vi "DSC Plotter.vi"() -> ()   [LabVIEW 2020]
uses:
  Time_Slot--Control.ctl
  <vilib>/lvdsc/historical/Read Traces (Numeric).vi
  <vilib>/lvdsc/NI_DSC.lvlib
  <vilib>/lvdsc/historical/Read Trace (Numeric).vi
  <userlib>/_OpenG.lib/array/array.llb/Index 1D Array Elements (String)__ogtk.vi
panel:
  in  "Tree":string[](tree)
  out "error out":errorcluster
  out "quality":i32[][](array[numeric])
  in  "options":T1={"interpolate data (F)"=TRUE, "extrapolate to now (F)"=FALSE, "remove data breaks (F)"=TRUE, "interpolation interval (1 s)"=1.0, "maintain trending info (T)"=FALSE} {"interpolation interval (1 s)" min=0.0 format="%0.2f"}
  out "empty?":bool
  out "Argument":string
  in  "Traces":T2(array[cluster])
  out "busy":bool
  out "Array 2":timestamp[](array[timestamp])
  out "Array":timestamp[](array[timestamp])
  out "time (s)":sgl
  out "Children Tags":string[](array[string])
  in  "Presets":u16(ring) items=["Select Preset", "Clear Chart", "Add New Preset"]
  in  "Tab Control":enum32{"Main", "Custom Time", "Settings"}(tab)
  in  "Time slots":T3=enum."8 Hours"
  in  "Seek Back Button":bool
  in  "Seek Forward Button":bool
  in  "Display Current":bool
  in  "time interval":T4 {"stop timestamp (now)" format="%<%X\n%x>T"; "start timestamp" format="%<%X\n%x>T"}
  in  "Display Chose Time Slot":bool
  in  "update rate(ms)":i32=10000
  in  "max points per trace (all)":i32=1000
  in  "OK":bool
  out "XY Graph":T5(graph)
  # "Time Window (drop down 1hr 1 day etc)\nchoose channel/s\npresets (inc time window and channels)\nExport to csv.\nLive mode return\nIf you select manual time interval shows that until live mode return button pressed\nwould be nice to have arrows to go back and forth in time."
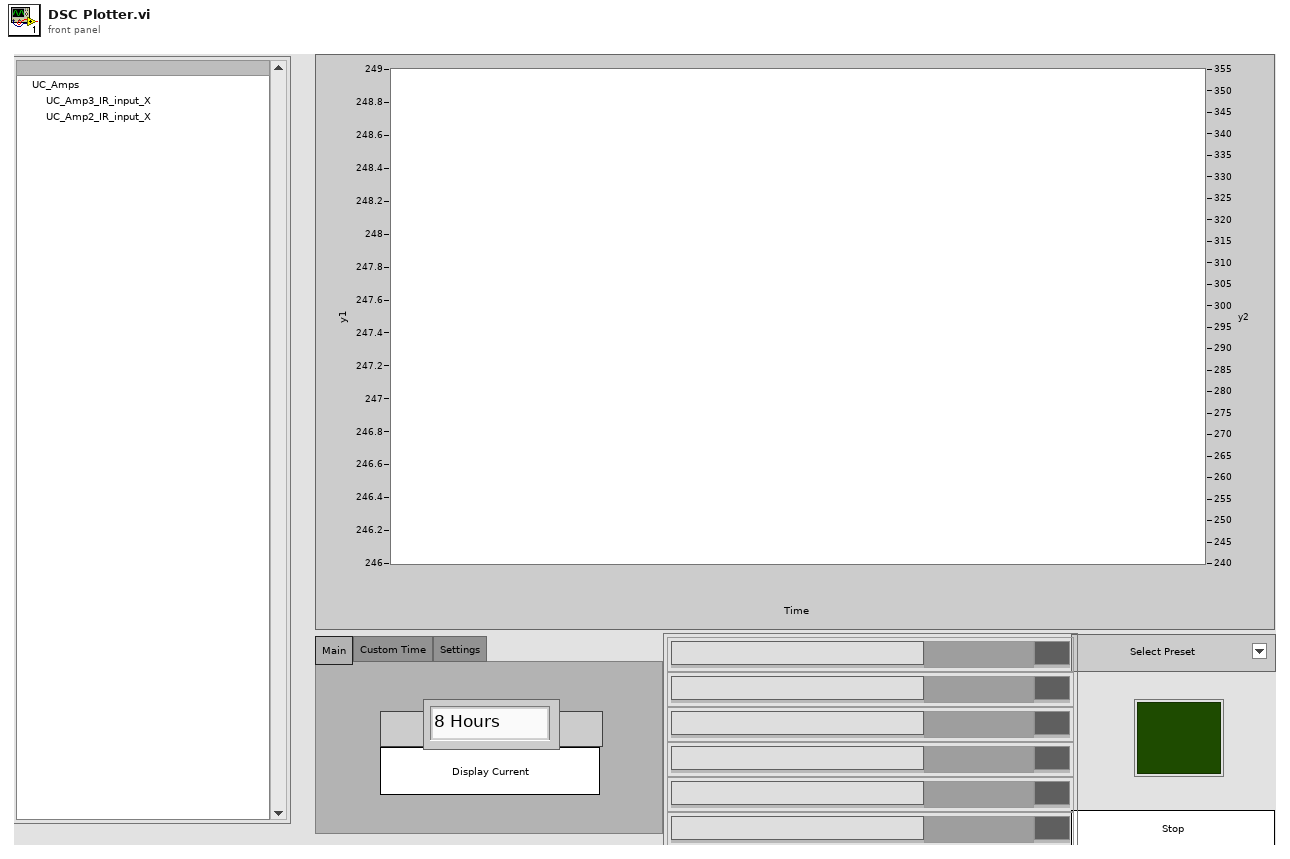
[diagram p1: front panel]
types:
  T1 = cluster{"interpolate data (F)":bool, "extrapolate to now (F)":bool, "remove data breaks (F)":bool, "interpolation interval (1 s)":dbl, "maintain trending info (T)":bool}
  T2 = cluster{"Name":string, "L/R scale":bool, "Color Box":u32}[]
  T3 = typedef "Time_Slot--Control.ctl" = enum16{"5 Mins", "15 Mins", "30 mins", "1 Hour", "8 Hours", "1 Day", "1 Week", "1 Month", "3 Months", "6 Months", "1 Year", "2 Years"}
  T4 = cluster{"start timestamp":timestamp, "stop timestamp (now)":timestamp}
  T5 = cluster{"timestamps":timestamp[], "data":dbl[]}[]
  T6 = cluster{"Name":string, "L/R scale":bool, "Color Box":u32}
  T7 = enum32{"invalid app kind", "Development System", "Run Time System", "Student Edition", "Embedded LabVIEW", "Evaluation", "Custom"}
  T8 = enum32{"Invalid", "Standard", "Closed", "Hidden", "Minimized", "Maximized"}
  T9 = cluster{"Core":cluster{"Current VI Reference":refnum<vi>, "Close Panel on Exit?":bool}, "options":cluster{"interpolate data (F)":bool, "extrapolate to now (F)":bool, "remove data breaks (F)":bool, "interpolation interval (1 s)":dbl, "maintain trending info (T)":bool}, "time interval":cluster{"start timestamp":timestamp, "stop timestamp (now)":timestamp}, "historical traces":cluster{"timestamps":timestamp[], "data":dbl[]}[], "Trace Names":string[], "max points per trace (all)":i32, "Time slots":T3, "Display Current Enable":bool, "update rate(ms)":i32, "All Traces from DB":string[], "Traces":cluster{"Name":string, "L/R scale":bool, "Color Box":u32}[]}
  T10 = typedef "mysql_authentication.ctl" = cluster{"User":string, "Password":string, "Database":string}
  T11 = cluster{"Port":u16, "IP Address":string, "Authentication":T10}
  T12 = cluster{"Current VI Reference":refnum<vi>, "Close Panel on Exit?":bool}
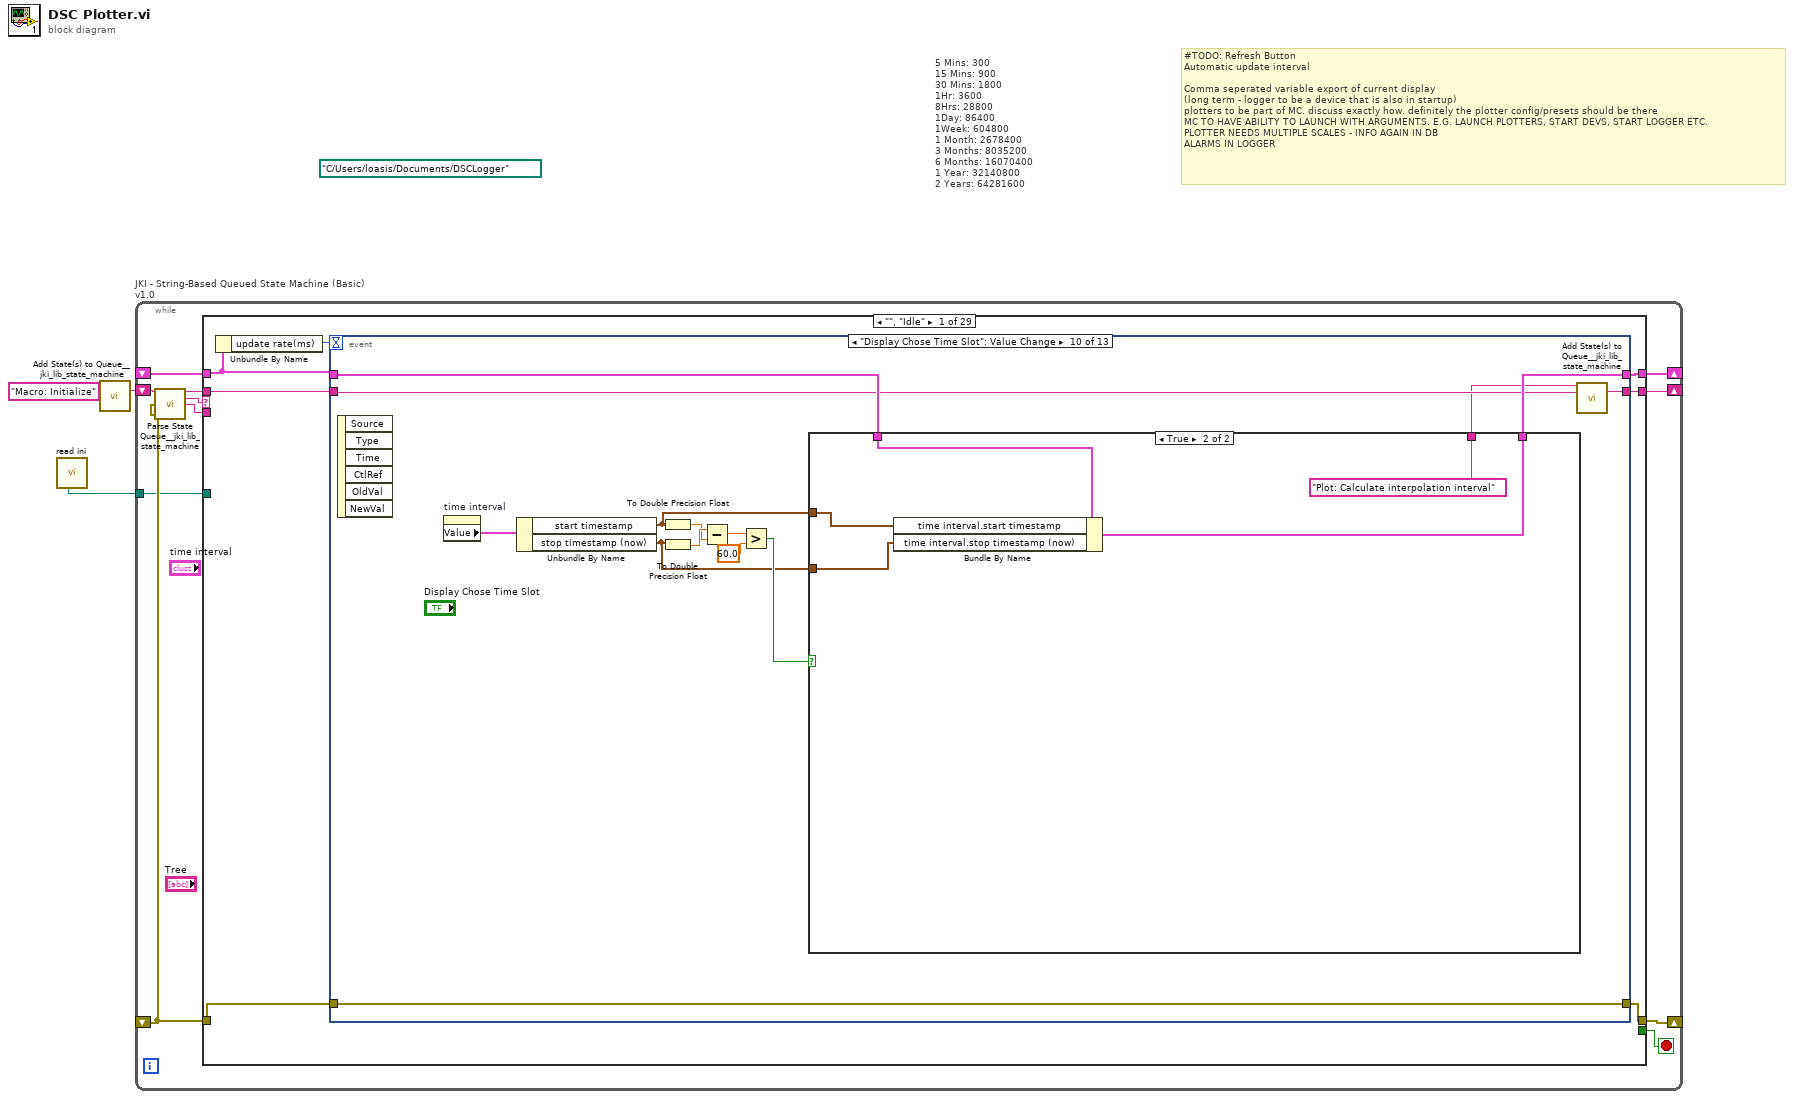
[diagram p0: block diagram]
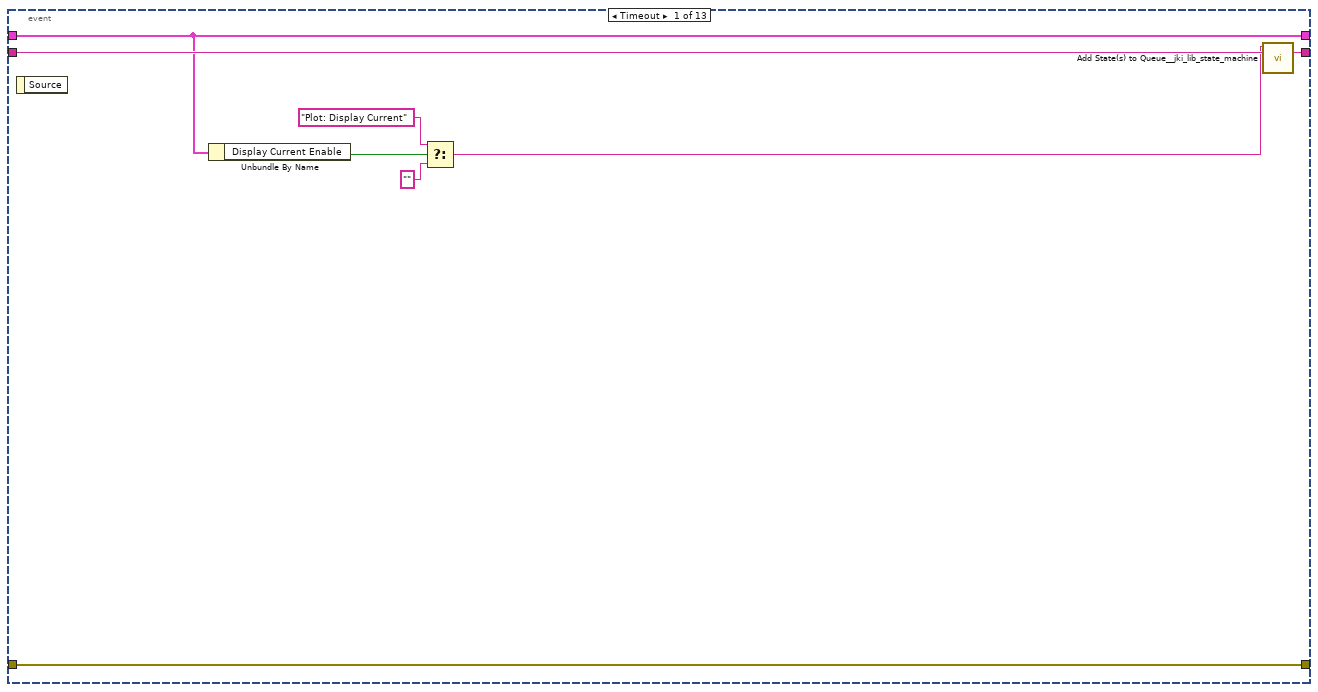
[diagram p2: hidden frame]
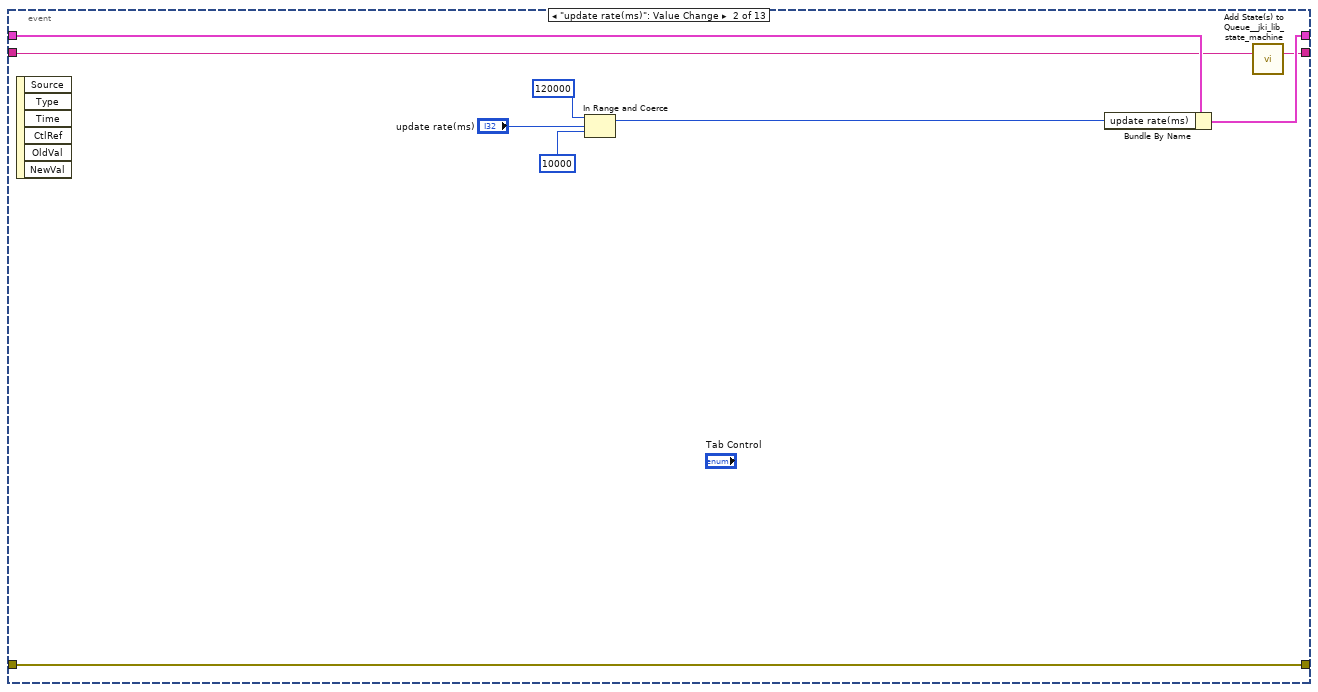
[diagram p3: hidden frame]
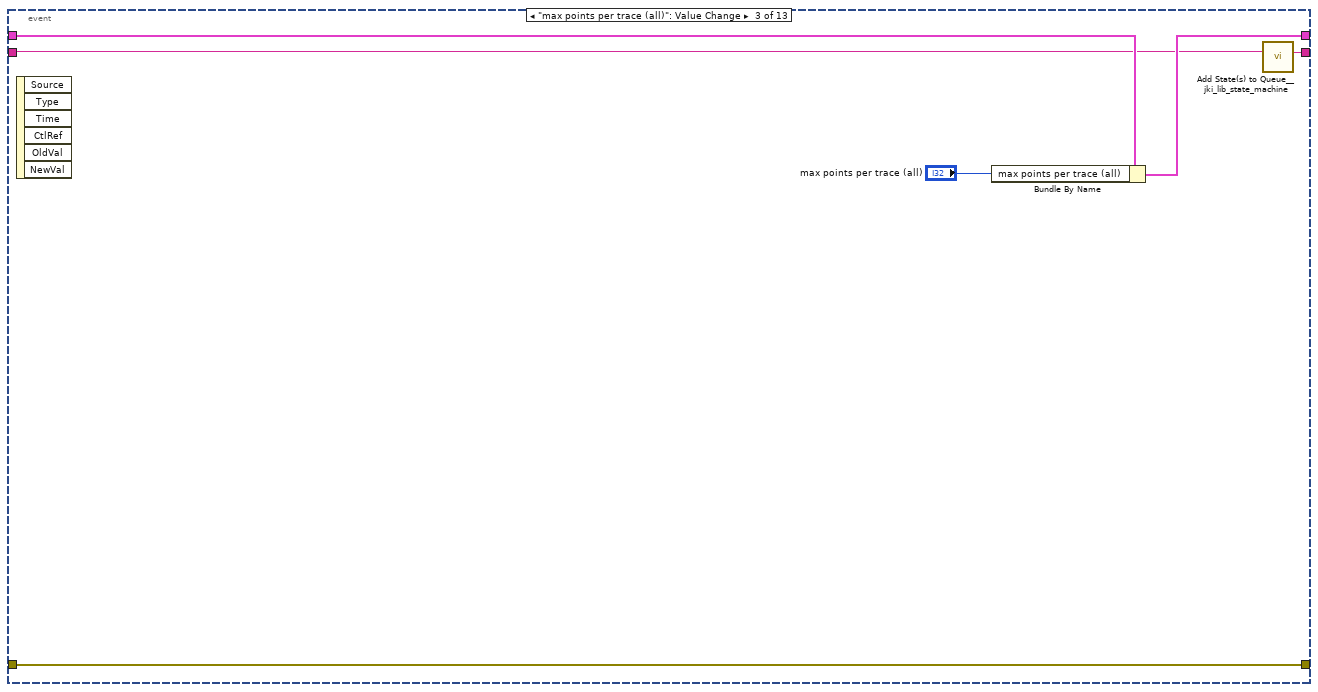
[diagram p4: hidden frame]
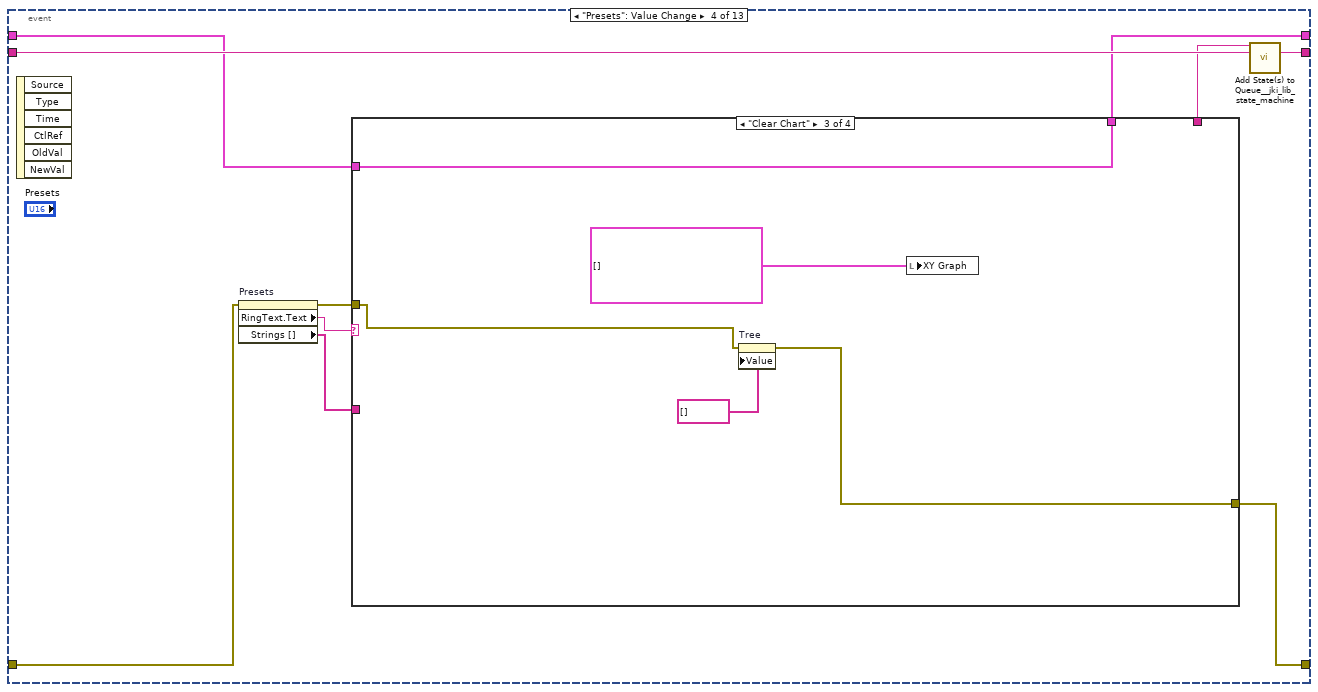
[diagram p5: hidden frame]
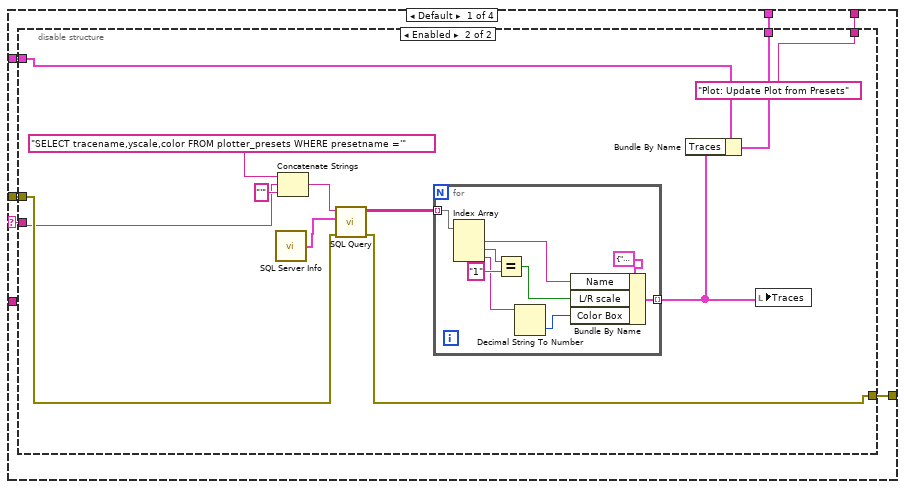
[diagram p6: hidden frame]
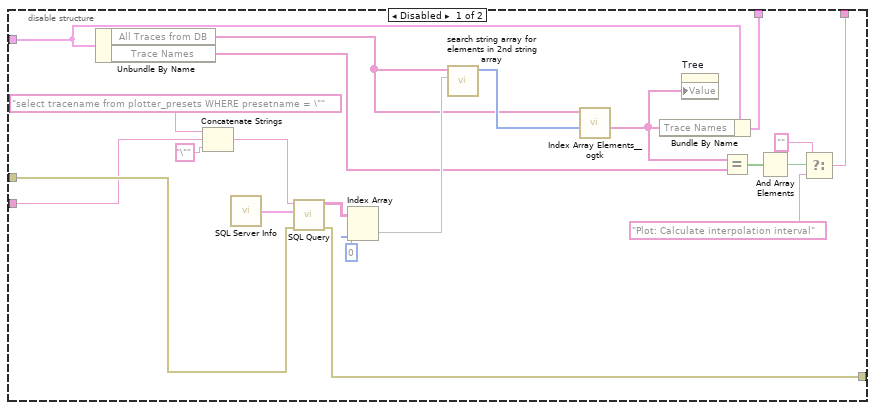
[diagram p7: hidden frame]
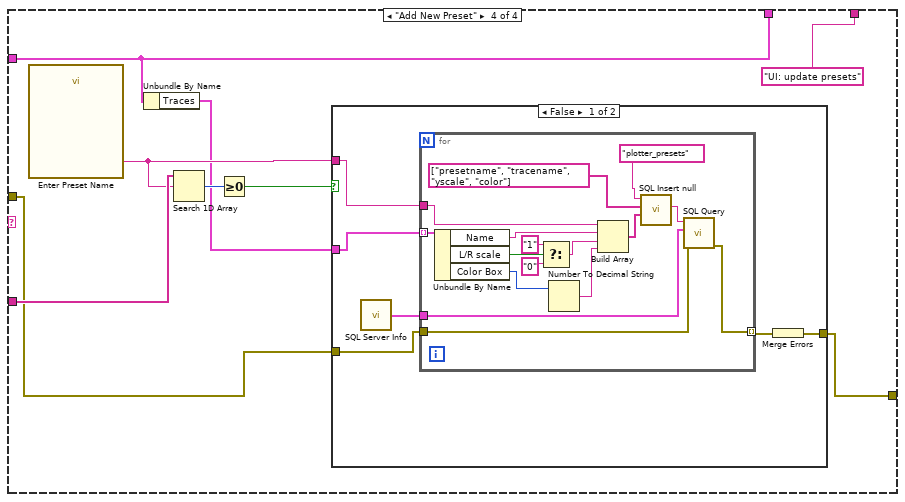
[diagram p9: hidden frame]
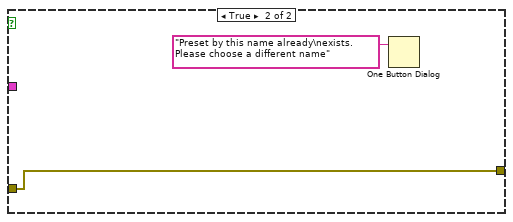
[diagram p10: hidden frame]
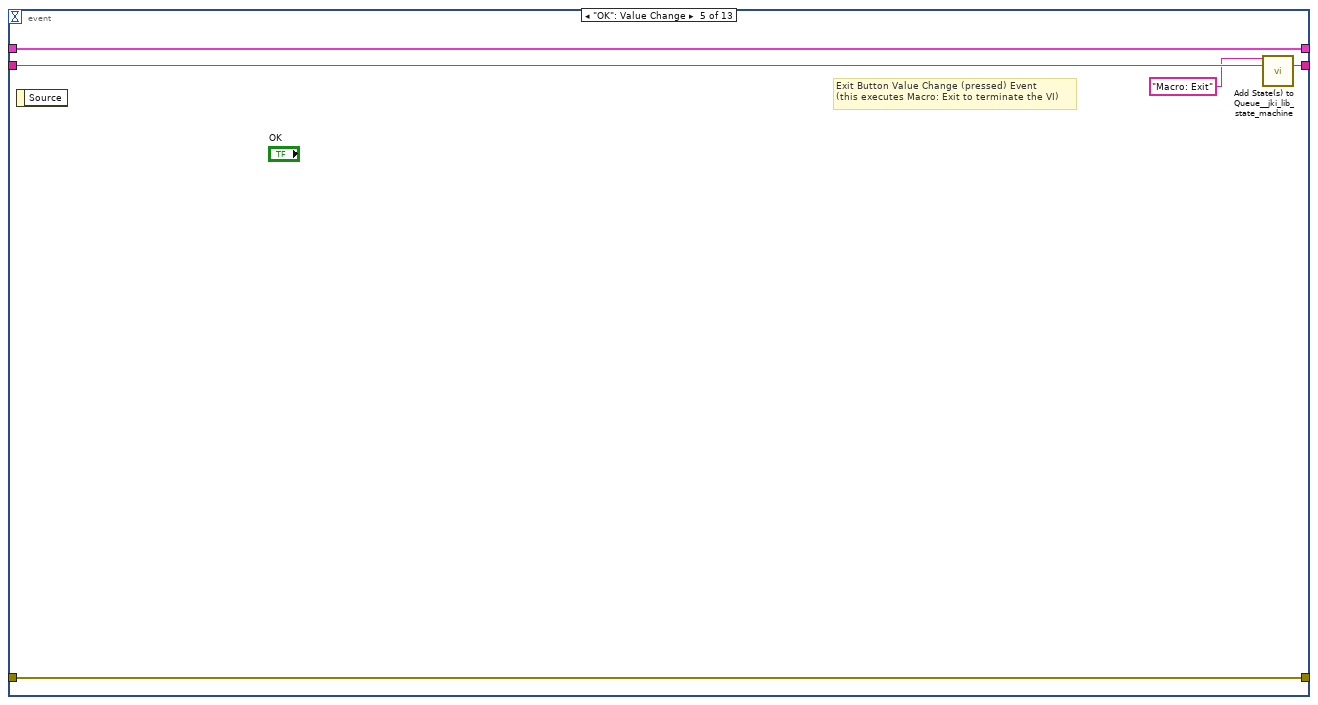
[diagram p11: hidden frame]
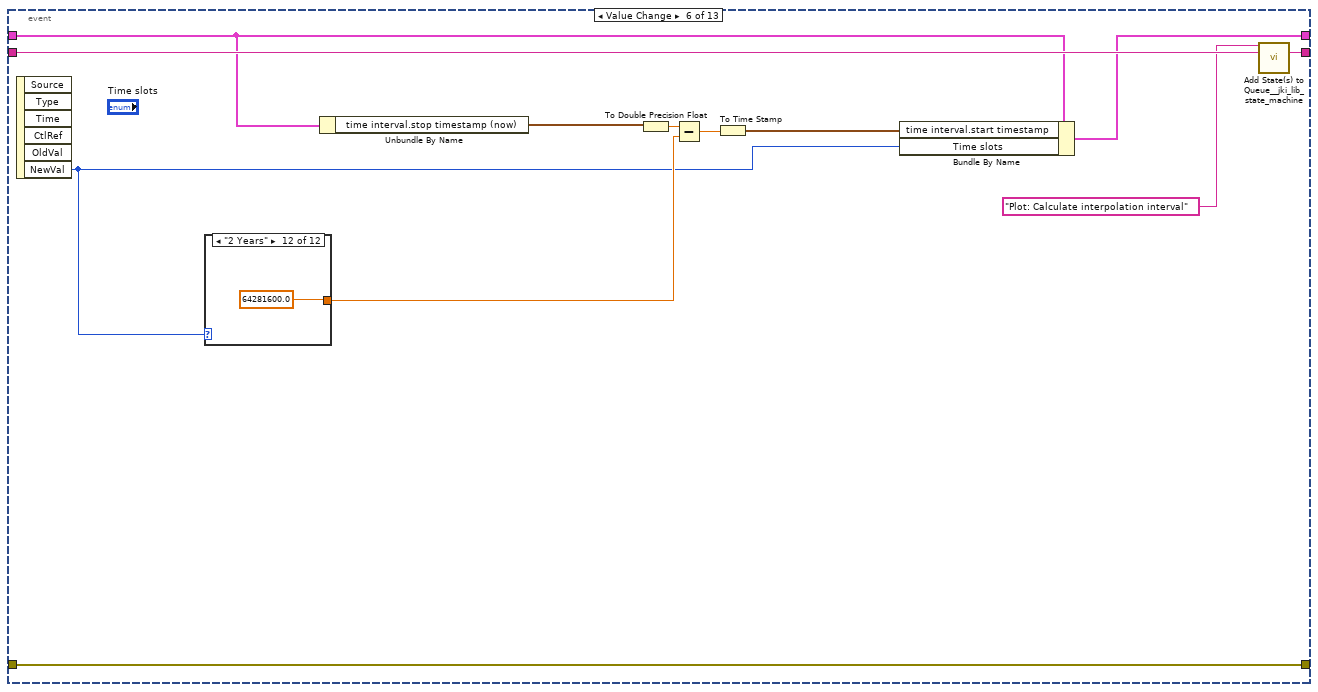
[diagram p12: hidden frame]
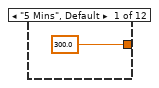
[diagram p13: hidden frame]
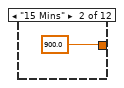
[diagram p14: hidden frame]
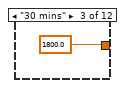
[diagram p15: hidden frame]
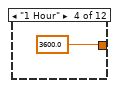
[diagram p16: hidden frame]
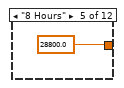
[diagram p17: hidden frame]
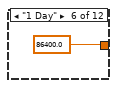
[diagram p18: hidden frame]
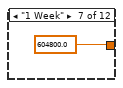
[diagram p19: hidden frame]
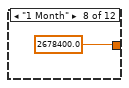
[diagram p20: hidden frame]
diagram:
  (unwired) path "C:/Users/loasis/Documents/DSCLogger" ("Application Directory")
  # "#TODO: Refresh Button\nAutomatic update interval\n\nComma seperated variable export of current display\n(long term - logger to be a device that is also in startup)\nplotters to be part of MC. discuss exactly how. definitely the plotter config/presets should be there\nMC TO HAVE ABILITY TO LAUNCH WITH ARGUMENTS. E.G. LAUNCH PLOTTERS, START DEVS, START LOGGER ETC.\nPLOTTER NEEDS MULTIPLE SCALES - INFO AGAIN IN DB\nALARMS IN LOGGER"
  # "5 Mins: 300\n15 Mins: 900\n30 Mins: 1800\n1Hr: 3600\n8Hrs: 28800\n1Day: 86400\n1Week: 604800\n1 Month: 2678400\n3 Months: 8035200\n6 Months: 16070400 \n1 Year: 32140800\n2 Years: 64281600"
  n1 = call "read ini.vi"() -> ("Database URL"=w1:path)  [unwired: 5 in, 6 out]
  n2 = call <vilib>:"Add State(s) to Queue__jki_lib_state_machine.vi"("State(s) in (\"\")"="Macro: Initialize") -> ("States Out"=w3:string)  [unwired: 14 in]
  n3 = while "JKI - String-Based Queued State Machine (Basic) v1.0" {
    shift-right: [w7] -> _
    shift-left: _ -> [w6]
    shift-right: [w10] -> _
    shift-left: _ -> [w5]
    shift-right: [w9] -> _
    shift-left: w3 -> [w11]
    tunnel: w1 -> [w4]
    stop <- w8 stop-if-true
    n4 = call <vilib>:"Parse State Queue__jki_lib_state_machine.vi"("State Queue"=w11, "Error In (no error)"=w5) -> ("Remaining States"=w13:string, "Current State"=w14:string, "Arguments"=w12:string)  [unwired: 11 in]
    n5 = case shown="\"\", \"Idle\"" w14 {
      selector: w14 -> [_ _ w348 _ _ _ _ _ _ _ _ _ _ _ _ _ _ _ _ _ _ _ _ _ _ _ _ _ _]
      tunnel: w13 -> [w21 w347 w352 w370 w376 w381 w385 w406 w412 w416 w431 w444 w472 w488 w499 w525 w530 w540 w544 w548 w553 w570 w579 w602 w623 w732 w749 w760 w770]
      tunnel: w12 -> [_ _ _ _ _ _ _ _ _ _ _ _ _ w483 w493 _ _ _ _ _ _ _ _ w589 w604 w726 _ _ _]
      tunnel: w6 -> [w16 w344 w350 w361 w373 w379 w382 _ w407 w413 w429 w442 w474 w486 w495 w522 w527 w537 w541 w545 w550 w566 w575 w595 w619 w730 w747 w758 w765]
      tunnel: [w19 w345 w354 w367 errorcluster {"status"=FALSE, "code"=0, "source"=""} ("error out") w378 w383 w403 w408 w414 w417 w432 w467 w484 w496 w523 w528 w538 w542 w546 w551 w568 w577 w600 w609 w729 w746 w752 w766] -> w10
      tunnel: w5 -> [w18 w345 w353 w367 w372 w378 w383 w403 w409 w414 w418 w433 w468 w485 w497 w523 w528 w538 w542 w546 w551 w568 w577 w600 w613 w729 w746 w753 w762]
      tunnel: [w20 w346 w351 w369 w375 w380 w384 w405 w411 w415 w430 w443 w473 w487 w498 w524 w529 w539 w543 w547 w552 w569 w578 w601 w622 w731 w748 w759 w769] -> w9
      tunnel: [_ _ _ _ _ TRUE _ _ _ _ _ _ _ _ _ _ _ _ _ _ _ _ _ _ _ _ _ _ _] -> w8
      tunnel: [w17 w344 w350 w368 w373 w379 w382 w404 w407 w413 w429 w442 w474 w486 w495 w522 w527 w537 w541 w545 w550 w565 w574 w594 w618 w730 w747 w757 w764] -> w7
      tunnel: w4 -> [_ _ _ _ _ _ _ _ _ _ _ _ _ _ _ _ _ _ _ _ _ _ _ _ w603 _ _ _ _]
      frame "", "Idle" {
        n6 = Unbundle By Name(w16) -> ("update rate(ms)"=w15:i32)
        n7 = event shown="[9] \"Display Chose Time Slot\": Value Change" {
          selector: _ -> [_ _ _ _ _ _ _ _ _ _ _ _ _]
          dyn-events: _ -> [_ _ _ _ _ _ _ _ _ _ _ _ _]
          timeout: w15 -> [_ _ _ _ _ _ _ _ _ _ _ _ _]
          tunnel: w21 -> [w29 w30 w39 w49 w147 w157 w174 w190 w209 w252 w285 w314 w343]
          tunnel: [w28 w31 w40 w50 w146 w158 w175 w191 w210 w253 w286 w315 w342] -> w20
          tunnel: w16 -> [w26 w37 w44 w48 w144 w153 w172 w183 w208 w257 w277 w306 w340]
          tunnel: [w27 w32 w41 w51 w145 w159 w176 w192 w211 w250 w287 w316 w341] -> w19
          tunnel: w18 -> [w27 w32 w41 w54 w145 w159 w176 w192 w211 w250 w287 w316 w341]
          tunnel: [w26 w38 w43 w47 w144 w152 w172 w189 w208 w254 w276 w305 w340] -> w17
          event Timeout {
            n8 = event-data() -> ()  [unwired: 1 in, 1 out]
            n9 = Unbundle By Name(w26) -> ("Display Current Enable"=w25:bool)
            n10 = Select(t="Plot: Display Current" ("State(s) in Front (\"\")"), s=w25, f="" ("State(s) in Front (\"\")")) -> (s? t:f=w23:string)
            n11 = call <vilib>:"Add State(s) to Queue__jki_lib_state_machine.vi"("State(s) in Front (\"\")"=w23, "State(s) in (\"\")"=w29) -> ("States Out"=w28:string)  [unwired: 13 in]
          }
          event "update rate(ms)": Value Change {
            n12 = event-data() -> ()  [unwired: 1 in, 6 out]
            n13 = In Range and Coerce(upper limit=120000, x="update rate(ms)", lower limit=10000) -> (coerced(x)=w33:i32)  [unwired: 1 out]
            n14 = Bundle By Name(cluster=w37, "update rate(ms)"=w33) -> (w38:T9)
            n15 = call <vilib>:"Add State(s) to Queue__jki_lib_state_machine.vi"("State(s) in (\"\")"=w30) -> ("States Out"=w31:string)  [unwired: 14 in]
          }
          event "max points per trace (all)": Value Change {
            n16 = event-data() -> ()  [unwired: 1 in, 6 out]
            n17 = Bundle By Name(cluster=w44, "max points per trace (all)"="max points per trace (all)") -> (w43:T9)
            n18 = call <vilib>:"Add State(s) to Queue__jki_lib_state_machine.vi"("State(s) in (\"\")"=w39) -> ("States Out"=w40:string)  [unwired: 14 in]
          }
          event "Presets": Value Change {
            n19 = event-data() -> ()  [unwired: 1 in, 6 out]
            n20 = property on="Presets" class="Ring (strict)"(error in=w54) -> (error out=w52:errorcluster, "RingText.Text"=w53:string, "Strings []"=w45:string[])  [unwired: 1 in, 1 out]
            n21 = case shown="\"Clear Chart\"" w53 {
              selector: w53 -> [w58 _ _ _]
              tunnel: w52 -> [w60 w103 w105 w114]
              tunnel: [w59 w103 w106 w113] -> w51
              tunnel: w48 -> [w57 w104 w109 w112]
              tunnel: [w56 w104 w109 w112] -> w47
              tunnel: [w55 _ _ "UI: update presets" ("t")] -> w46
              tunnel: w45 -> [_ _ _ w118]
              frame Default {
                n22 = disable-structure shown="Enabled" {
                  disable-tunnel: w60 -> [w80 w88]
                  disable-tunnel: [w79 w87] -> w59
                  disable-tunnel: w58 -> [w78 w86]
                  disable-tunnel: w57 -> [w69 w84]
                  disable-tunnel: [w68 w85] -> w56
                  disable-tunnel: [w62 "Plot: Update Plot from Presets" ("t")] -> w55
                  frame Disabled {
                    n23 = Unbundle By Name(w69) -> ("All Traces from DB"=w70:string[], "Trace Names"=w67:string[])
                    n24 = Concatenate Strings("select tracename from plotter_presets WHERE presetname = \"", w78, "\"" ("string")) -> (w76:string)
                    n25 = call "SQL Server Info.vi"() -> ("SQL Server Info"=w81:T11)
                    n26 = call "SQL Query.vi"("error in (no error)"=w80, "SQL Server Info"=w81, "Query"=w76) -> ("error out"=w79:errorcluster, "data"=w74:string[][])  [unwired: 7 in]
                    n27 = Index Array(array=w74, index (col)=0 ("index (row)")) -> (element=w72:string[])  [unwired: 1 in]
                    n28 = call "search string array for elements in 2nd string array.vi"("search for"=w72, "search in"=w70) -> ("Indices of Elements"=w71:i32[])  [unwired: 9 in]
                    n29 = call-poly <userlib>:"Index Array Elements__ogtk.vi"("indices"=w71, "array"=w70) -> ("elements"=w61:string[])  [unwired: 9 in]
                    n30 = Bundle By Name(cluster=w69, "Trace Names"=w61) -> (w68:T9)
                    n31 = property on="Tree" class="Tree (strict)"("Value"=w61) -> ()  [unwired: 2 in, 2 out]
                    n32 = Equal?(x=w61, y=w67) -> (x = y?=w66:bool[])
                    n33 = And Array Elements(Boolean array=w66) -> (logical AND=w65:bool)
                    n34 = Select(t="", s=w65, f="Plot: Calculate interpolation interval") -> (s? t:f=w62:string)
                  }
                  frame Enabled {
                    n35 = call "SQL Server Info.vi"() -> ("SQL Server Info"=w91:T11)
                    n36 = Concatenate Strings("SELECT tracename,yscale,color FROM plotter_presets WHERE presetname ='" ("Query"), w86, "'" ("string")) -> (w93:string)
                    n37 = call "SQL Query.vi"("error in (no error)"=w88, "SQL Server Info"=w91, "Query"=w93) -> ("error out"=w87:errorcluster, "data"=w89:string[][])  [unwired: 7 in]
                    n38 = for {
                      tunnel: w89 -> [w101] mode=indexing
                      tunnel: [w94] -> w83 mode=indexing
                      n39 = Index Array(array=w101) -> (element #1=w100:string, element #2=w99:string, element #3=w95:string)  [unwired: 3 in]
                      n40 = Equal?(x=w99, y="1") -> (x = y?=w97:bool)
                      n41 = Decimal String To Number(string=w95) -> (number=w96:i32)  [unwired: 2 in, 1 out]
                      n42 = Bundle By Name(cluster=T6 {"Name"="", "L/R scale"=FALSE, "Color Box"=0} ("Trace cluster"), "Name"=w100, "L/R scale"=w97, "Color Box"=w96) -> (w94:T6)
                    }
                    n43 = Bundle By Name(cluster=w84, "Traces"=w83) -> (w85:T9)
                    n44 = local write "Traces"(w83) -> ()
                  }
                }
              }
              frame "Select Preset" {
              }
              frame "Clear Chart" {
                n45 = property on="Tree" class="Tree (strict)"(error in=w105, "Value"=string[] [] ("Tree")) -> (error out=w106:errorcluster)  [unwired: 1 in, 1 out]
                n46 = local write "XY Graph"(T5 [] ("XY Graph")) -> ()
              }
              frame "Add New Preset" {
                n47 = call "Enter Preset Name"() -> ("Preset Name"=w115:string)  [unwired: 17 in, 2 out]
                n48 = Unbundle By Name(w112) -> ("Traces"=w111:T2)
                n49 = Search 1D Array(1D array=w118, element=w115) -> (index of element=w117:i32)  [unwired: 1 in]
                n50 = Greater Or Equal To 0?(x=w117) -> (x >= 0?=w116:bool)
                n51 = case shown="False" w116 {
                  tunnel: w111 -> [w123 _]
                  tunnel: w115 -> [w122 _]
                  tunnel: w114 -> [w121 w141]
                  tunnel: [w119 w141] -> w113
                  frame False {
                    n52 = call "SQL Server Info.vi"() -> ("SQL Server Info"=w124:T11)
                    n53 = for {
                      tunnel: w124 -> [w140]
                      tunnel: w123 -> [w132] mode=indexing
                      tunnel: w122 -> [w135]
                      tunnel: w121 -> [w134]
                      tunnel: [w133] -> w120 mode=indexing
                      n54 = Unbundle By Name(w132) -> ("Name"=w131:string, "L/R scale"=w130:bool, "Color Box"=w126:u32)
                      n55 = Select(t="1", s=w130, f="0") -> (s? t:f=w127:string)
                      n56 = Number To Decimal String(number=w126) -> (decimal integer string=w125:string)  [unwired: 1 in]
                      n57 = Build Array(w135, w131, w127, w125) -> (w136:string[])
                      n58 = call "SQL Insert null.vi"("Values"=w136, "Column Names"=string[] ["presetname", "tracename", "yscale", "color"], "Table"="plotter_presets") -> ("Query String"=w139:string)  [unwired: 8 in]
                      n59 = call "SQL Query.vi"("error in (no error)"=w134, "SQL Server Info"=w140, "Query"=w139) -> ("error out"=w133:errorcluster)  [unwired: 7 in, 1 out]
                    }
                    n60 = Merge Errors(w120) -> (w119:errorcluster)
                  }
                  frame True {
                    n61 = One Button Dialog(message="Preset by this name already\nexists. Please choose a different name") -> ()  [unwired: 1 in, 1 out]
                  }
                }
              }
            }
            n62 = call <vilib>:"Add State(s) to Queue__jki_lib_state_machine.vi"("State(s) in Front (\"\")"=w46, "State(s) in (\"\")"=w49) -> ("States Out"=w50:string)  [unwired: 13 in]
          }
          event "OK": Value Change {
            # "Exit Button Value Change (pressed) Event\n(this executes Macro: Exit to terminate the VI)"
            n63 = event-data() -> ()  [unwired: 1 in, 1 out]
            n64 = call <vilib>:"Add State(s) to Queue__jki_lib_state_machine.vi"("State(s) in Front (\"\")"="Macro: Exit", "State(s) in (\"\")"=w147) -> ("States Out"=w146:string)  [unwired: 13 in]
          }
          event Value Change {
            n65 = event-data() -> ("NewVal"=w148:T3)  [unwired: 1 in, 5 out]
            n66 = case shown="\"2 Years\"" w148 {
              tunnel: [300.0 ("y") 900.0 ("y") 1800.0 ("y") 3600.0 ("y") 28800.0 ("y") 86400.0 ("y") 604800.0 ("y") 2678400.0 ("y") 8035200.0 ("y") 16070400.0 ("y") 32140800.0 ("y") 64281600.0 ("y")] -> w154
              frame "5 Mins", Default {
              }
              frame "15 Mins" {
              }
              frame "30 mins" {
              }
              frame "1 Hour" {
              }
              frame "8 Hours" {
              }
              frame "1 Day" {
              }
              frame "1 Week" {
              }
              frame "1 Month" {
              }
              frame "3 Months" {
              }
              frame "6 Months" {
              }
              frame "1 Year" {
              }
              frame "2 Years" {
              }
            }
            n67 = Unbundle By Name(w153) -> ("time interval.stop timestamp (now)"=w155:timestamp)
            n68 = To Double Precision Float(number=w155) -> (double precision float=w156:dbl)
            n69 = Subtract(x=w156, y=w154) -> (x-y=w151:dbl)
            n70 = To Time Stamp(1:w151) -> (0:w150:timestamp)
            n71 = Bundle By Name(cluster=w153, "time interval.start timestamp"=w150, "Time slots"=w148) -> (w152:T9)
            n72 = call <vilib>:"Add State(s) to Queue__jki_lib_state_machine.vi"("State(s) in Front (\"\")"="Plot: Calculate interpolation interval" ("State(s) in Front (\"\")"), "State(s) in (\"\")"=w157) -> ("States Out"=w158:string)  [unwired: 13 in]
          }
          event "Display Current": Value Change {
            n73 = event-data() -> ()  [unwired: 1 in, 6 out]
            n74 = call <vilib>:"Add State(s) to Queue__jki_lib_state_machine.vi"("State(s) in Front (\"\")"="Plot: Display Current" ("State(s) in Front (\"\")"), "State(s) in (\"\")"=w174) -> ("States Out"=w175:string)  [unwired: 13 in]
          }
          event "Tree": Value Change {
            (unwired) "\\\\192.168.14.132\\Belladata\\LASERBAY-DEV\\Logger Master\\"
            (unwired) "\\\\192.168.14.132\\Logger Master\\"
            n75 = event-data() -> ("NewVal"=w184:string[])  [unwired: 1 in, 5 out]
            n76 = Array Size(array=w184) -> (size(s)=w187:i32)
            n77 = Greater?(x=w187, y=6) -> (0:w186:bool)
            n78 = case shown="True" w186 {
              tunnel: w184 -> [w196 w198]
              tunnel: [w196 w197] -> w180
              frame False {
              }
              frame True {
                n79 = Array Subset(array=w198, length=6) -> (w197:string[])  [unwired: 1 in]
                n80 = property on="Tree" class="Tree (strict)"("Value"=w197) -> ()  [unwired: 2 in, 2 out]
              }
            }
            n81 = disable-structure shown="Enabled" {
              disable-tunnel: w180 -> [w201 w204]
              disable-tunnel: [w200 w204] -> w182
              frame Disabled {
                n82 = for {
                  tunnel: w201 -> [w202] mode=indexing
                  tunnel: [w202] -> w200 mode=indexing
                  n83 = Concatenate Strings("\\\\LASERBAY-DEV\\Logger Master\\", w202) -> ()  [unwired: 1 out]
                }
              }
              frame Enabled {
              }
            }
            n84 = Array Size(array=w180) -> (size(s)=w179:i32)
            n85 = Initialize Array(T6 {"Name"="", "L/R scale"=FALSE, "Color Box"=0} ("Trace cluster"), w179) -> (w178:T2)
            n86 = for {
              tunnel: w182 -> [w194] mode=indexing
              tunnel: w178 -> [w195] mode=indexing
              tunnel: [w193] -> w177 mode=indexing
              n87 = Bundle By Name(cluster=w195, "Name"=w194) -> (w193:T6)
            }
            n88 = Bundle By Name(cluster=w183, "Trace Names"=w182, "Traces"=w177) -> (w189:T9)
            n89 = call <vilib>:"Add State(s) to Queue__jki_lib_state_machine.vi"("State(s) in Front (\"\")"="Plot: Calculate interpolation interval" ("State(s) in Front (\"\")"), "State(s) in (\"\")"=w190) -> ("States Out"=w191:string)  [unwired: 13 in]
          }
          event "Traces": Value Change {
            n90 = event-data() -> ("OldVal"=w207:T2, "NewVal"=w206:T2)  [unwired: 1 in, 4 out]
            n91 = for {
              tunnel: w207 -> [w224] mode=indexing
              tunnel: w206 -> [w223] mode=indexing
              tunnel: w206 -> [w215]
              i -> [w214]
              n92 = Unbundle By Name(w223) -> ("Name"=w217:string, "L/R scale"=w221:bool, "Color Box"=w220:u32)
              n93 = Unbundle By Name(w224) -> ("Name"=w218:string, "L/R scale"=w222:bool, "Color Box"=w219:u32)
              n94 = Equal?(x=w219, y=w220) -> (x = y?=w212:bool)
              n95 = Equal?(x=w222, y=w221) -> (x = y?=w216:bool)
              n96 = Equal?(x=w218, y=w217) -> (x = y?=w213:bool)
              n97 = case shown="True" w213 {
                tunnel: w216 -> [_ w228]
                tunnel: w215 -> [_ w227]
                tunnel: w214 -> [_ w226]
                tunnel: w212 -> [_ w225]
                frame False {
                }
                frame True {
                  n98 = stacked-sequence {
                    tunnel: w228 -> [w231 _]
                    tunnel: w227 -> [w230 w242]
                    tunnel: w226 -> [w229 w241]
                    tunnel: w225 -> [_ w243]
                    frame #0 {
                      n99 = case shown="False" w231 {
                        tunnel: w230 -> [w239 _]
                        tunnel: w229 -> [w233 _]
                        frame False {
                          (unwired) u8 2 ("Y Scale.Scale Fit")
                          n100 = Index Array(array=w239, index=w233) -> (element=w238:T6)
                          n101 = Unbundle By Name(w238) -> ("L/R scale"=w237:bool)
                          n102 = To Unsigned Long Integer(number=w233) -> (unsigned 32bit integer=w232:u32)
                          n103 = Select(t=u32 1 ("f"), s=w237, f=u32 0) -> (s? t:f=w235:u32)
                          n104 = control-ref of="XY Graph"() -> (w240:refnum<vi>)
                          n105 = property class="XYGraph (strict)"(reference=w240, "Active Plot"=w232, "Plot.YScaleIdx"=w235) -> ()  [unwired: 1 in, 2 out]
                        }
                        frame True {
                        }
                      }
                    }
                    frame #1 {
                      n106 = case shown="False" w243 {
                        tunnel: w242 -> [w246 _]
                        tunnel: w241 -> [w245 _]
                        frame False {
                          n107 = Index Array(array=w246, index=w245) -> (element=w248:T6)
                          n108 = Unbundle By Name(w248) -> ("Color Box"=w244:u32)
                          n109 = To Unsigned Long Integer(number=w245) -> (unsigned 32bit integer=w247:u32)
                          n110 = control-ref of="XY Graph"() -> (w249:refnum<vi>)
                          n111 = property class="XYGraph (strict)"(reference=w249, "Active Plot"=w247, "Plot.Plot Color"=w244) -> ()  [unwired: 1 in, 2 out]
                        }
                        frame True {
                        }
                      }
                    }
                  }
                }
              }
            }
            n112 = call <vilib>:"Add State(s) to Queue__jki_lib_state_machine.vi"("State(s) in Front (\"\")"="Plot: Display Data" ("State(s) in Front (\"\")"), "State(s) in (\"\")"=w209) -> ("States Out"=w210:string)  [unwired: 13 in]
          }
          event "Display Chose Time Slot": Value Change {
            n113 = event-data() -> ()  [unwired: 1 in, 6 out]
            n114 = property on="time interval" class="Clust (strict)"() -> ("Value"=w263:T4)  [unwired: 2 in, 2 out]
            n115 = Unbundle By Name(w263) -> ("start timestamp"=w256:timestamp, "stop timestamp (now)"=w255:timestamp)
            n116 = To Double Precision Float(number=w256) -> (double precision float=w261:dbl)
            n117 = To Double Precision Float(number=w255) -> (double precision float=w262:dbl)
            n118 = Subtract(x=w262, y=w261) -> (x-y=w260:dbl)
            n119 = Greater?(x=w260, y=60.0) -> (0:w258:bool)
            n120 = case shown="True" w258 {
              tunnel: w257 -> [w265 w270]
              tunnel: w256 -> [_ w269]
              tunnel: w255 -> [_ w268]
              tunnel: [w265 w267] -> w254
              tunnel: ["" "Plot: Calculate interpolation interval" ("State(s) in Front (\"\")")] -> w251
              frame False {
              }
              frame True {
                n121 = Bundle By Name(cluster=w270, "time interval.start timestamp"=w269, "time interval.stop timestamp (now)"=w268) -> (w267:T9)
              }
            }
            n122 = call <vilib>:"Add State(s) to Queue__jki_lib_state_machine.vi"("State(s) in Front (\"\")"=w251, "State(s) in (\"\")"=w252) -> ("States Out"=w253:string)  [unwired: 13 in]
          }
          event "Seek Back Button": Value Change {
            n123 = event-data() -> ()  [unwired: 1 in, 6 out]
            n124 = Unbundle By Name(w277) -> ("Time slots"=w283:T3)
            n125 = case shown="\"15 Mins\"" w283 {
              tunnel: [300.0 ("y") 900.0 ("y") 1800.0 ("y") 3600.0 ("y") 28800.0 ("y") 86400.0 ("y") 604800.0 ("y") 2678400.0 ("y") 8035200.0 ("y") 16070400.0 ("y") 32140800.0 ("y") 64281600.0 ("y")] -> w278
              frame "5 Mins", Default {
              }
              frame "15 Mins" {
              }
              frame "30 mins" {
              }
              frame "1 Hour" {
              }
              frame "8 Hours" {
              }
              frame "1 Day" {
              }
              frame "1 Week" {
              }
              frame "1 Month" {
              }
              frame "3 Months" {
              }
              frame "6 Months" {
              }
              frame "1 Year" {
              }
              frame "2 Years" {
              }
            }
            n126 = Unbundle By Name(w277) -> ("time interval.start timestamp"=w281:timestamp, "time interval.stop timestamp (now)"=w279:timestamp)
            n127 = To Double Precision Float(number=w281) -> (double precision float=w282:dbl)
            n128 = To Double Precision Float(number=w279) -> (double precision float=w280:dbl)
            n129 = Subtract(x=w282, y=w278) -> (x-y=w275:dbl)
            n130 = Subtract(x=w280, y=w278) -> (x-y=w272:dbl)
            n131 = To Time Stamp(1:w275) -> (0:w274:timestamp)
            n132 = To Time Stamp(1:w272) -> (0:w273:timestamp)
            n133 = Bundle By Name(cluster=w277, "time interval.start timestamp"=w274, "time interval.stop timestamp (now)"=w273, "Display Current Enable"=FALSE) -> (w276:T9)
            n134 = call <vilib>:"Add State(s) to Queue__jki_lib_state_machine.vi"("State(s) in Front (\"\")"="Plot: Calculate interpolation interval" ("State(s) in Front (\"\")"), "State(s) in (\"\")"=w285) -> ("States Out"=w286:string)  [unwired: 13 in]
          }
          event "Seek Forward Button": Value Change {
            n135 = event-data() -> ()  [unwired: 1 in, 6 out]
            n136 = Unbundle By Name(w306) -> ("Time slots"=w312:T3)
            n137 = case shown="\"2 Years\"" w312 {
              tunnel: [300.0 ("y") 900.0 ("y") 1800.0 ("y") 3600.0 ("y") 28800.0 ("y") 86400.0 ("y") 604800.0 ("y") 2678400.0 ("y") 8035200.0 ("y") 16070400.0 ("y") 32140800.0 ("y") 64281600.0 ("y")] -> w307
              frame "5 Mins", Default {
              }
              frame "15 Mins" {
              }
              frame "30 mins" {
              }
              frame "1 Hour" {
              }
              frame "8 Hours" {
              }
              frame "1 Day" {
              }
              frame "1 Week" {
              }
              frame "1 Month" {
              }
              frame "3 Months" {
              }
              frame "6 Months" {
              }
              frame "1 Year" {
              }
              frame "2 Years" {
              }
            }
            n138 = Unbundle By Name(w306) -> ("time interval.start timestamp"=w310:timestamp, "time interval.stop timestamp (now)"=w308:timestamp)
            n139 = Get Date/Time In Seconds() -> (seconds since 1Jan1904=w303:timestamp)
            n140 = To Double Precision Float(number=w303) -> (double precision float=w301:dbl)
            n141 = To Double Precision Float(number=w310) -> (double precision float=w311:dbl)
            n142 = To Double Precision Float(number=w308) -> (double precision float=w309:dbl)
            n143 = Add(x=w311, y=w307) -> (x+y=w304:dbl)
            n144 = Add(x=w309, y=w307) -> (x+y=w302:dbl)
            n145 = Greater?(x=w302, y=w301) -> (0:w300:bool)
            n146 = case shown="True" w300 {
              tunnel: ["Plot: Calculate interpolation interval" ("State(s) in Front (\"\")") "Plot: Display Current" ("State(s) in Front (\"\")")] -> w313
              tunnel: w306 -> [w322 w324]
              tunnel: [w321 w324] -> w305
              tunnel: w304 -> [w320 _]
              tunnel: w302 -> [w317 _]
              frame False {
                n147 = To Time Stamp(1:w320) -> (0:w319:timestamp)
                n148 = To Time Stamp(1:w317) -> (0:w318:timestamp)
                n149 = Bundle By Name(cluster=w322, "time interval.start timestamp"=w319, "time interval.stop timestamp (now)"=w318) -> (w321:T9)
              }
              frame True {
              }
            }
            n150 = call <vilib>:"Add State(s) to Queue__jki_lib_state_machine.vi"("State(s) in Front (\"\")"=w313, "State(s) in (\"\")"=w314) -> ("States Out"=w315:string)  [unwired: 13 in]
          }
          event Panel Close? {
            # "Discard the event because we'll close the front panel ourselves in Macro: Exit"
            # "Close Panel button (pressed) Event\n(this executes Macro: Exit to terminate the VI)"
            n151 = event-data() -> ()  [unwired: 1 in, 1 out]
            n152 = event-data("Discard?"=TRUE) -> ()  [unwired: 1 in, 1 out]
            n153 = call <vilib>:"Add State(s) to Queue__jki_lib_state_machine.vi"("State(s) in Front (\"\")"="Macro: Exit", "State(s) in (\"\")"=w343) -> ("States Out"=w342:string)  [unwired: 13 in]
          }
        }
      }
      frame "---------- Core ----------" {
        # "Do not put any code in this frame.\n(it is a separator no-op)"
        n154 = call <vilib>:"Add State(s) to Queue__jki_lib_state_machine.vi"("State(s) in (\"\")"=w347) -> ("States Out"=w346:string)  [unwired: 14 in]
      }
      frame Default {
        w357 = 42 items=["No error", "Argument error", "Memory is full", "Out of zone", "End of file", "File already open", "Generic file I/O error", "File not found", "File permission error", "Disk is full", "Duplicate path", "Too many files open", "System feature not enabled", "Resource file not found", "Cannot add resource", "Resource not found", "Image not found", "Image memory error", "Pen does not exist", "Config type invalid", "Config token not found", "Config parse error", "Config memory error", "Bad external code format", "Bad external code offset", "External code not present", "Null window", "Destroy window error", "Null menu", "Print aborted", "Bad print record", "Print driver error", "Windows error during printing", "Memory error during printing", "Print dialog error", "Generic print error", "Invalid device refnum", "Device not found", "Device parameter error", "Device unit error", "Cannot open device", "Device call aborted", "Generic error", "Cancelled by user", "Object ID too low", "Object ID too high", "Object not in heap", "Unknown heap", "Unknown object (invalid DefProc)", "Unknown object (DefProc not in table)", "Message out of range", "Invalid (null) method", "Unknown message", "Manager call not supported", "Bad address", "Network operation in progress", "Network operation timed out", "Connection is busy", "Network attribute not supported", "Network error", "Address in use", "System out of memory", "Connection aborted", "Connection refused", "Not connected", "Already connected", "Connection closed", "Initialization error (interapplication manager)", "Bad occurrence", "Wait on unbound occurrence handler", "Occurrence queue overflow", "Datalog type conflict", "Unused", "Unrecognized type (interapplication manager)", "Memory corrupt", "Failed to make temporary DLL", "Old CIN version", "Drag socket not found", "Failed to load drop-object", "Failed to register OLE object", "Failed to release OLE object", "Format specifier type mismatch", "Unknown format specifier", "Too few format specifiers", "Too many format specifiers", "Scan failed", "Newer CIN version", "Error converting to variant", "Runtime menu error", "Password tampered", "Variant attribute not found", "Incompatible variant data type", "Event data is not available", "Event Store is not present", "Occurrence is not found", "Event Queue is not created", "Event info is not available", "Refnum passed is NULL", "Error retrieving Class GUID", "Error retrieving CoClass GUID", "Error retrieving TypeLib GUID.", "Bad built application magic bytes.", "Specific driver is different from the specific driver associated with the Logical Name.", "There is no session opened to the class driver.", "Max Error", "MAX - Error with config objects", "MAX - Error loading configuration", "MAX - Group not supported"]
        # "Current State"
        # "Do not delete, rename, or modify this frame.\n(this is used to capture unhandled states and typos)"
        # "Handle mistyped state name (developer tool)"
        n155 = Format Into String(format string="Software Exception: Unhandled State \"%s\"." ("message"), error in=w353, w348) -> (resulting string=w356:string, error out=w355:errorcluster)  [unwired: 1 in]
        n156 = call <vilib>:"Error Cluster From Error Code.vi"("show call chain? (False)"=TRUE, "error in (no error)"=w355, "error message (\"\")"=w356, "error code (0)"=w357) -> ("error out"=w354:errorcluster)  [unwired: 5 in]
        n157 = call <vilib>:"Add State(s) to Queue__jki_lib_state_machine.vi"("State(s) in (\"\")"=w352) -> ("States Out"=w351:string)  [unwired: 14 in]
      }
      frame "Initialize Core Data" {
        # "Do not delete, rename, or modify this frame.\n(this is used to determine panel behavior on exit)"
        # "originally closed?"
        # "exe?"
        # "If panel starts closed or is an EXE, then close it when we exit"
        n158 = property class="VI"() -> ("Front Panel.Open"=w366:bool)  [unwired: 2 in, 2 out]
        n159 = property class="App"() -> ("App.Kind"=w365:T7)  [unwired: 2 in, 2 out]
        n160 = control-ref of="Current VI Reference"() -> (w359:refnum<vi>)
        n161 = Not(x=w366) -> (.not. x?=w363:bool)
        n162 = Equal?(x=w365, y=T7."Run Time System" ("Application:Kind")) -> (x = y?=w362:bool)
        n163 = Or(x=w363, y=w362) -> (x .or. y?=w360:bool)
        n164 = Bundle By Name(cluster=w361, "Core.Current VI Reference"=w359, "Core.Close Panel on Exit?"=w360) -> (w368:T9)
        n165 = call <vilib>:"Add State(s) to Queue__jki_lib_state_machine.vi"("State(s) in (\"\")"=w370) -> ("States Out"=w369:string)  [unwired: 14 in]
      }
      frame "Error Handler" {
        # "Unhandled Error -- Display it"
        # "Handle any errors here.\nYou can also output any states to clean-up after errors occur"
        # "Clear error"
        n166 = call <vilib>:"General Error Handler.vi"("error in (no error)"=w372) -> ()  [unwired: 10 in, 5 out]
        n167 = call <vilib>:"Add State(s) to Queue__jki_lib_state_machine.vi"("State(s) in Front (\"\")"="/* Post Error States", "State(s) in (\"\")"=w376) -> ("States Out"=w375:string)  [unwired: 13 in]
      }
      frame "Exit" {
        # "Do not put any code in this frame.\n(No errors that occur here will be handled.)"
        n168 = call <vilib>:"Add State(s) to Queue__jki_lib_state_machine.vi"("State(s) in (\"\")"=w381) -> ("States Out"=w380:string)  [unwired: 14 in]
      }
      frame "---------- Data ----------" {
        # "Do not put any code in this frame.\n(It is a separator no-op. You can make a copy of this frame to create a new Data frame)"
        n169 = call <vilib>:"Add State(s) to Queue__jki_lib_state_machine.vi"("State(s) in (\"\")"=w385) -> ("States Out"=w384:string)  [unwired: 14 in]
      }
      frame "Data: Initialize" {
        w386 = T2 []  # Traces
        w387 = string[] []  # All Traces from DB
        w388 = 1000  # max points per trace (all)
        w389 = 60000  # update rate(ms)
        w390 = T4 {"start timestamp"=timestamp(0 s since 1904-01-01), "stop timestamp (now)"=timestamp(0 s since 1904-01-01)}  # time interval
        w391 = TRUE  # Display Current Enable
        w392 = Time_Slot--Control."8 Hours"  # Time slots
        w399 = string[] []  # Trace Names
        w400 = T5 []  # historical traces
        w402 = T12 {"Current VI Reference"=refnum, "Close Panel on Exit?"=FALSE}  # Core
        # "8 Hrs"
        n170 = Get Date/Time In Seconds() -> (seconds since 1Jan1904=w395:timestamp)
        n171 = To Double Precision Float(number=w395) -> (double precision float=w397:dbl)
        n172 = Subtract(x=w397, y=28800.0) -> (x-y=w396:dbl)
        n173 = To Time Stamp(1:w396) -> (0:w393:timestamp)
        n174 = Bundle By Name(cluster=w390, "stop timestamp (now)"=w395, "start timestamp"=w393) -> (w398:T4)
        n175 = property on="Time slots" class="Enum (strict)"("Value"=w392) -> ()  [unwired: 2 in, 2 out]
        n176 = Bundle("Core"=w402, "options"="options", "time interval"=w398, "historical traces"=w400, "Trace Names"=w399, "max points per trace (all)"=w388, "Time slots"=w392, "Display Current Enable"=w391, "update rate(ms)"=w389, "All Traces from DB"=w387, "Traces"=w386) -> (w404:T9)  [unwired: 1 in]
        n177 = call <vilib>:"Add State(s) to Queue__jki_lib_state_machine.vi"("State(s) in (\"\")"=w406) -> ("States Out"=w405:string)  [unwired: 14 in]
      }
      frame "Data: Cleanup" {
        # "Cleanup any data and references, here.\n(this is called automatically, by the Macro: Exit)"
        n178 = Unbundle By Name(w407) -> ("Core.Current VI Reference"=w410:refnum<vi>)
        n179 = Close Reference(reference=w410, error in (no error)=w409) -> (error out=w408:errorcluster)
        n180 = call <vilib>:"Add State(s) to Queue__jki_lib_state_machine.vi"("State(s) in (\"\")"=w412) -> ("States Out"=w411:string)  [unwired: 14 in]
      }
      frame "---------- UI ----------" {
        # "Do not put any code in this frame.\n(It is a separator no-op. You can make a copy of this frame to create a new UI frame)"
        n181 = call <vilib>:"Add State(s) to Queue__jki_lib_state_machine.vi"("State(s) in (\"\")"=w416) -> ("States Out"=w415:string)  [unwired: 14 in]
      }
      frame "UI: update presets" {
        # "Do not put any code in this frame.\n(It is a separator no-op. You can make a copy of this frame to create a new UI frame)"
        n182 = call "SQL Server Info.vi"() -> ("SQL Server Info"=w426:T11)
        n183 = call "SQL Query.vi"("error in (no error)"=w418, "SQL Server Info"=w426, "Query"="SELECT DISTINCT presetname FROM plotter_presets") -> ("error out"=w419:errorcluster, "data"=w428:string[][])  [unwired: 7 in]
        n184 = Index Array(array=w428, index (col)=0 ("disabled index (col)")) -> (element=w422:string[])  [unwired: 1 in]
        n185 = Insert Into Array(array=string[] ["Select Preset", "Clear Chart", "Add New Preset"], index=2, new element=w422) -> (w421:string[])
        n186 = property on="Presets" class="Ring (strict)"(error in=w419, "Strings []"=w421, "Value"=0) -> (error out=w417:errorcluster)  [unwired: 1 in, 1 out]
        n187 = call <vilib>:"Add State(s) to Queue__jki_lib_state_machine.vi"("State(s) in (\"\")"=w431) -> ("States Out"=w430:string)  [unwired: 14 in]
      }
      frame "UI: Initialize" {
        # "Initialize the User Interface, here.\n(this is called automatically, by the Macro: Init)"
        n188 = invoke on="Tree" class="Tree (strict)" method="Reinit To Default"() -> (error out=w434:errorcluster)  [unwired: 3 in, 2 out]
        n189 = call "SQL Server Info.vi"() -> ("SQL Server Info"=w441:T11)
        n190 = call "SQL Query.vi"("error in (no error)"=w433, "SQL Server Info"=w441, "Query"="SELECT DISTINCT channel_group FROM logger") -> ("error out"=w432:errorcluster, "data"=w436:string[][])  [unwired: 7 in]
        n191 = invoke on="Tree" class="Tree (strict)" method="Edit Tree Items.Delete"(error in=w434, "Delete Children"=TRUE ("Delete Children?")) -> (error out=w440:errorcluster)  [unwired: 3 in, 4 out]
        n192 = Index Array(array=w436, index (col)=0 ("disabled index (col)")) -> (element=w438:string[])  [unwired: 1 in]
        n193 = for {
          tunnel: w438 -> [w446] mode=indexing
          tunnel: w440 -> [w452]
          tunnel: w441 -> [w451]
          n194 = invoke on="Tree" class="Tree (strict)" method="Edit Tree Items.Add Item"(error in=w452, "Child Position"=-1 ("Child Posn"), "Left Cell"=w446, "Child Only?"=FALSE) -> (error out=w447:errorcluster)  [unwired: 5 in, 8 out]
          n195 = Concatenate Strings("SELECT device,variable,alias FROM logger WHERE channel_group ='" ("Query"), w446, "'" ("string")) -> (w448:string)
          n196 = call "SQL Query.vi"("error in (no error)"=w447, "SQL Server Info"=w451, "Query"=w448) -> ("data"=w445:string[][])  [unwired: 7 in, 1 out]
          n197 = for {
            tunnel: w446 -> [w464]
            tunnel: w445 -> [w463] mode=indexing
            n198 = Index Array(array=w463) -> (element #1=w455:string, element #2=w457:string, element #3=w459:string)  [unwired: 3 in]
            n199 = Empty String/Path?(string/path=w459) -> (empty?=w462:bool)
            n200 = Concatenate Strings(w455, " " ("string"), w457) -> (w458:string)
            n201 = Select(t=w458, s=w462, f=w459) -> (s? t:f=w460:string)
            n202 = invoke on="Tree" class="Tree (strict)" method="Edit Tree Items.Add Item"("Parent Tag"=w464, "Left Cell"=w460, "Child Tag"=w460, "Child Only?"=TRUE) -> ()  [unwired: 5 in, 9 out]
          }
        }
        n203 = call <vilib>:"Add State(s) to Queue__jki_lib_state_machine.vi"("State(s) in (\"\")"=w444) -> ("States Out"=w443:string)  [unwired: 14 in]
      }
      frame "UI: Get Tree Items" {
        n204 = control-ref of="Tree"() -> (w471:refnum<vi>)
        n205 = call "getchildren.vi"("Tree Reference In"=w471) -> ("Children Tags"=w470:string[], "Tree Reference Out"=w469:refnum<vi>)  [unwired: 2 in, 1 out]
        n206 = for {
          tunnel: w470 -> [w480] mode=indexing
          shift-right: [w481] -> _
          shift-left: w469 -> [w482]
          tunnel: w468 -> [w479]
          tunnel: [w478] -> w467
          shift-right: [w476] -> w466
          shift-left: string[] [] -> [w475]
          n207 = call "getchildren.vi"("error in (no error)"=w479, "Parent Tag"=w480, "Tree Reference In"=w482) -> ("error out"=w478:errorcluster, "Children Tags"=w477:string[], "Tree Reference Out"=w481:refnum<vi>)
          n208 = Build Array (concatenate)(w475, w477) -> (w476:string[])
        }
        "Children Tags" <- w466
        n209 = call <vilib>:"Add State(s) to Queue__jki_lib_state_machine.vi"("State(s) in (\"\")"=w472) -> ("States Out"=w473:string)  [unwired: 14 in]
      }
      frame "UI: Cursor Set" {
        # "Argument"
        # "Set and Unset Cursor Busy.\n(Usage: \"UI: Cursor Set >> Busy|Idle\")"
        n210 = case shown="\"Idle\", Default" w483 {
          tunnel: w485 -> [w490 w492]
          tunnel: [w489 w491] -> w484
          frame "Idle", Default {
            n211 = call <vilib>:"Unset Busy.vi"("error in (no error)"=w490) -> ("error out"=w489:errorcluster)  [unwired: 10 in]
          }
          frame "Busy" {
            n212 = call <vilib>:"Set Busy.vi"("error in (no error)"=w492) -> ("error out"=w491:errorcluster)  [unwired: 9 in, 1 out]
          }
        }
        n213 = call <vilib>:"Add State(s) to Queue__jki_lib_state_machine.vi"("State(s) in (\"\")"=w488) -> ("States Out"=w487:string)  [unwired: 14 in]
      }
      frame "UI: Front Panel State" {
        # "Argument"
        # "Set Front Panel Open or Closed\n(Usage: \"UI: Front Panel State >> Open|Close\")"
        n214 = Unbundle By Name(w495) -> ("Core.Current VI Reference"=w494:refnum<vi>)
        n215 = case shown="\"Open\", Default" w493 {
          tunnel: w497 -> [w503 w516]
          tunnel: [w505 w517] -> w496
          tunnel: w494 -> [w504 w514]
          frame "Open", Default {
            n216 = property class="VI"(reference=w504, error in=w503) -> (reference out=w501:refnum<vi>, error out=w502:errorcluster, "Front Panel.Open"=w500:bool)
            n217 = case shown="False" w500 {
              tunnel: [w508 w511] -> w505
              tunnel: w502 -> [w507 w511]
              tunnel: w501 -> [w506 _]
              frame False {
                n218 = invoke class="VI" method="FP.Open"(reference=w506, error in=w507, "Activate"=TRUE, "State"=T8."Standard") -> (error out=w508:errorcluster)  [unwired: 1 in, 4 out]
              }
              frame True {
              }
            }
          }
          frame "Close" {
            n219 = property class="VI"(reference=w514, error in=w516) -> (reference out=w513:refnum<vi>, error out=w515:errorcluster, "Front Panel.Open"=w512:bool)
            n220 = case shown="True" w512 {
              tunnel: [w518 w521] -> w517
              tunnel: w515 -> [w518 w520]
              tunnel: w513 -> [_ w519]
              frame False {
              }
              frame True {
                n221 = invoke class="VI" method="FP.Close"(reference=w519, error in=w520) -> (error out=w521:errorcluster)  [unwired: 1 in, 2 out]
              }
            }
          }
        }
        n222 = call <vilib>:"Add State(s) to Queue__jki_lib_state_machine.vi"("State(s) in (\"\")"=w499) -> ("States Out"=w498:string)  [unwired: 14 in]
      }
      frame "---------- Macro ----------" {
        # "Do not put any code in this frame.\n(It is a separator no-op. You can make a copy of this frame to create a new Macro frame)"
        n223 = call <vilib>:"Add State(s) to Queue__jki_lib_state_machine.vi"("State(s) in (\"\")"=w525) -> ("States Out"=w524:string)  [unwired: 14 in]
      }
      frame "Macro: Initialize" {
        w526 = "Data: Initialize\nInitialize Core Data\nUI: Initialize\nUI: update presets\nUI: Front Panel State >> Open\nUI: Get Tree Items\nMISC: get preset from arguments"  # Data: Initialize Initialize Core Data UI: Initialize UI: update presets UI: Front Panel State >> Open UI: Get Tree Items MISC: get preset from arguments
        # "Initialization Macro\n(This is called once, when the VI starts)"
        n224 = call <vilib>:"Add State(s) to Queue__jki_lib_state_machine.vi"("State(s) in Front (\"\")"=w526, "State(s) in (\"\")"=w530) -> ("States Out"=w529:string)  [unwired: 13 in]
      }
      frame "Macro: Exit" {
        # "Exit Macro\n(This is called once, when the VI exits)"
        n225 = Unbundle By Name(w537) -> ("Core.Close Panel on Exit?"=w536:bool)
        n226 = Select(t="UI: Front Panel State >> Close", s=w536, f="") -> (s? t:f=w533:string)
        n227 = call <vilib>:"Add State(s) to Queue__jki_lib_state_machine.vi"("State(s) in (\"\")"=w533, "State(s) at Back (\"\")"="Data: Cleanup\nExit") -> ("States Out"=w531:string)  [unwired: 13 in]
        n228 = call <vilib>:"Add State(s) to Queue__jki_lib_state_machine.vi"("State(s) in Front (\"\")"=w531, "State(s) in (\"\")"=w540) -> ("States Out"=w539:string)  [unwired: 13 in]
      }
      frame "---------- Data Query ----------" {
        # "Template Separator\n(You can make a copy of, or modify, this frame)"
        n229 = call <vilib>:"Add State(s) to Queue__jki_lib_state_machine.vi"("State(s) in (\"\")"=w544) -> ("States Out"=w543:string)  [unwired: 14 in]
      }
      frame "----------------Traces----------------" {
        # "Template Separator\n(You can make a copy of, or modify, this frame)"
        n230 = call <vilib>:"Add State(s) to Queue__jki_lib_state_machine.vi"("State(s) in (\"\")"=w548) -> ("States Out"=w547:string)  [unwired: 14 in]
      }
      frame "MISC: get preset from arguments" {
        # "Template Separator\n(You can make a copy of, or modify, this frame)"
        n231 = disable-structure "Factory Pattern: Enable plugin" shown="RUN_TIME_ENGINE==True" {
          disable-tunnel: [_ ""] -> w549
          frame condition #0 (active) {
          }
          frame condition #1 {
            n232 = control-ref of="This Application"() -> (w561:refnum<vi>)
            n233 = property class="App"(reference=w561) -> ("App.Args"=w559:string[])  [unwired: 1 in, 2 out]
            n234 = Index Array(array=w559, index=1) -> (element=w556:string)
            "Argument" <- w556
            n235 = property on="Presets" class="Ring (strict)"() -> ("Strings []"=w557:string[])  [unwired: 2 in, 2 out]
            n236 = Search 1D Array(1D array=w557, element=w556) -> (index of element=w555:i32)  [unwired: 1 in]
            n237 = Greater Or Equal To 0?(x=w555) -> (x >= 0?=w554:bool)
            n238 = case shown="True" w554 {
              tunnel: w555 -> [_ w562]
              frame False {
              }
              frame True {
                n239 = property on="Presets" class="Ring (strict)"("Val(Sgnl)"=w562) -> ()  [unwired: 2 in, 2 out]
              }
            }
          }
        }
        n240 = call <vilib>:"Add State(s) to Queue__jki_lib_state_machine.vi"("State(s) in Front (\"\")"=w549, "State(s) in (\"\")"=w553) -> ("States Out"=w552:string)  [unwired: 13 in]
      }
      frame "Plot: Update Plot from Presets" {
        n241 = Unbundle By Name(w566) -> ("Traces"=w567:T2)
        n242 = for {
          tunnel: w567 -> [w572] mode=indexing
          tunnel: [w571] -> w563 mode=indexing
          n243 = Unbundle By Name(w572) -> ("Name"=w571:string)
        }
        n244 = property on="Tree" class="Tree (strict)"("Value"=w563) -> ()  [unwired: 2 in, 2 out]
        n245 = Bundle By Name(cluster=w566, "Trace Names"=w563) -> (w565:T9)
        n246 = call <vilib>:"Add State(s) to Queue__jki_lib_state_machine.vi"("State(s) in Front (\"\")"="Plot: Calculate interpolation interval>>preset" ("State(s) in Front (\"\")"), "State(s) in (\"\")"=w570) -> ("States Out"=w569:string)  [unwired: 13 in]
      }
      frame "Traces: update cluster" {
        # "Template Separator\n(You can make a copy of, or modify, this frame)"
        n247 = Unbundle By Name(w575) -> ("Traces"=w576:T2)
        n248 = for {
          tunnel: w576 -> [w583] mode=indexing
          tunnel: [w580] -> w573 mode=indexing
          i -> [w585]
          n249 = control-ref of="XY Graph"() -> (w586:refnum<vi>)
          n250 = property class="XYGraph (strict)"(reference=w586, "Active Plot"=w585) -> ("Plot.YScaleIdx"=w584:u32, "Plot.Plot Color"=w581:u32)  [unwired: 1 in, 2 out]
          n251 = Not Equal To 0?(x=w584) -> (x != 0?=w582:bool)
          n252 = Bundle By Name(cluster=w583, "L/R scale"=w582, "Color Box"=w581) -> (w580:T6)
        }
        n253 = Bundle By Name(cluster=w575, "Traces"=w573) -> (w574:T9)
        n254 = local write "Traces"(w573) -> ()
        n255 = call <vilib>:"Add State(s) to Queue__jki_lib_state_machine.vi"("State(s) in (\"\")"=w579) -> ("States Out"=w578:string)  [unwired: 14 in]
      }
      frame "Plot: Calculate interpolation interval" {
        n256 = Unbundle By Name(w595) -> ("time interval.stop timestamp (now)"=w597:timestamp, "time interval.start timestamp"=w596:timestamp, "max points per trace (all)"=w592:i32)
        n257 = To Double Precision Float(number=w597) -> (double precision float=w598:dbl)
        n258 = To Double Precision Float(number=w596) -> (double precision float=w599:dbl)
        n259 = Subtract(x=w598, y=w599) -> (x-y=w593:dbl)
        n260 = Divide(x=w593, y=w592) -> (x/y=w591:dbl)
        n261 = Format Into String(format string="Plot: Query Data>>%s", w589) -> (resulting string=w587:string)  [unwired: 2 in, 1 out]
        n262 = Round To Nearest(number=w591) -> (nearest integer value=w590:dbl)
        n263 = Bundle By Name(cluster=w595, "options.interpolation interval (1 s)"=w590) -> (w594:T9)
        n264 = call <vilib>:"Add State(s) to Queue__jki_lib_state_machine.vi"("State(s) in Front (\"\")"=w587, "State(s) in (\"\")"=w602) -> ("States Out"=w601:string)  [unwired: 13 in]
      }
      frame "Plot: Query Data" {
        n265 = Unbundle By Name(w619) -> ("max points per trace (all)"=w617:i32, "Trace Names"=w620:string[], "time interval"=w615:T4, "options"=w614:T1)
        n266 = property on="time interval" class="Clust (strict)"("Value"=w615) -> ()  [unwired: 2 in, 2 out]
        n267 = property on="options" class="Clust (strict)"("Value"=w614) -> ()  [unwired: 2 in, 2 out]
        n268 = Empty Array?(array=w620) -> (empty?=w621:bool)
        n269 = call <userlib>:"Tick Count (ms)__ogtk.vi"("error in (no error)"=w613) -> ("error out"=w612:errorcluster, "millisecond timer value"=w608:u32)  [unwired: 9 in]
        n270 = case shown="False" w621 {
          tunnel: w620 -> [w631 _]
          tunnel: w615 -> [w640 _]
          tunnel: w612 -> [w644 w722]
          tunnel: [w641 w722] -> w611
          tunnel: w614 -> [w639 _]
          tunnel: w619 -> [w643 w723]
          tunnel: [w642 w723] -> w618
          tunnel: w617 -> [w632 _]
          tunnel: [w625 _] -> w616
          tunnel: w604 -> [w626 _]
          tunnel: w603 -> [w624 _]
          frame False {
            n271 = First Call?() -> (First Call?: T/F=w636:bool)
            n272 = case shown="False" w636 {
              tunnel: [w713 30 ("timeout (30 s)")] -> w633
              tunnel: w631 -> [w719 _]
              frame False {
                n273 = Array Size(array=w719) -> (size(s)=w718:i32)
                n274 = Multiply(x=w718, y=3 ("timeout (30 s)")) -> (x*y=w716:i32)
                n275 = In Range and Coerce(upper limit=10, x=w716, lower limit=1) -> (coerced(x)=w713:i32)  [unwired: 1 out]
              }
              frame True {
              }
            }
            n276 = local read "empty?"() -> (w629:bool)
            n277 = case shown="True" w629 {
              tunnel: w624 -> [w645 w656]
              tunnel: w631 -> [_ w655]
              tunnel: w633 -> [_ w654]
              tunnel: w632 -> [_ w653]
              tunnel: [w645 w646] -> w628
              frame False {
              }
              frame True {
                n278 = Get Date/Time In Seconds() -> (seconds since 1Jan1904=w649:timestamp)
                n279 = To Double Precision Float(number=w649) -> (double precision float=w650:dbl)
                n280 = To Double Precision Float(number=w649) -> (double precision float=w652:dbl)
                n281 = Subtract(x=w650, y=900.0) -> (x-y=w659:dbl)
                n282 = Subtract(x=w652, y=30.0) -> (x-y=w648:dbl)
                n283 = To Time Stamp(1:w659) -> (0:w661:timestamp)
                n284 = To Time Stamp(1:w648) -> (0:w647:timestamp)
                n285 = local write "busy"(FALSE ("busy")) -> ()
                n286 = Bundle(w661, w647) -> (w657:cluster{timestamp, timestamp})  [unwired: 1 in]
                n287 = call-poly <vilib>:"Read Traces.vi"("timeout (30 s)"=w654, "max points per trace (all)"=w653, "time interval"=w657, "trace names"=w655, "database URL"=w656) -> ("database URL out"=w646:path)  [unwired: 3 in, 3 out]
              }
            }
            n288 = disable-structure shown="Enabled" {
              disable-tunnel: w631 -> [w673 w697]
              disable-tunnel: w628 -> [w672 w698]
              disable-tunnel: w640 -> [w671 w704]
              disable-tunnel: w639 -> [w670 w702]
              disable-tunnel: w632 -> [w669 w701]
              disable-tunnel: [w668 w695] -> w638
              disable-tunnel: [w666 w703] -> w637
              disable-tunnel: w633 -> [w665 w700]
              disable-tunnel: [w664 w699] -> w634
              disable-tunnel: [_ w694] -> w630
              frame Disabled {
                n289 = for {
                  tunnel: w673 -> [w681] mode=indexing
                  tunnel: w672 -> [w685]
                  tunnel: w671 -> [w683]
                  tunnel: w670 -> [w682]
                  tunnel: [w680] -> w664 mode=indexing
                  tunnel: [w679] -> w668 mode=indexing
                  tunnel: w669 -> [w674]
                  workers-P: 8 -> [_]
                  tunnel: [w678] -> w666
                  tunnel: w665 -> [w677]
                  tunnel: [w676] -> w662 mode=indexing
                  tunnel: [w675] -> w663 mode=indexing
                  n290 = disable-structure shown="Enabled" {
                    disable-tunnel: w685 -> [w692 w693]
                    disable-tunnel: [w690 _] -> w676
                    disable-tunnel: [w689 _] -> w675
                    disable-tunnel: [w688 w693] -> w684
                    disable-tunnel: w681 -> [w687 _]
                    frame Enabled {
                      n291 = call <vilib>:"Get Trace Info.vi"("timeout (30 s)"=5, "trace name"=w687, "database URL"=w692) -> ("error out"=w686:errorcluster, "last timestamp"=w689:timestamp, "first timestamp"=w690:timestamp, "database URL out"=w688:path)  [unwired: 4 in, 1 out]
                      n292 = call <vilib>:"Clear Errors.vi"("error in (no error)"=w686) -> ()  [unwired: 5 in, 2 out]
                    }
                    frame Disabled {
                    }
                  }
                  n293 = call-poly <vilib>:"Read Trace.vi"("options"=w682, "timeout (30 s)"=w677, "max points per trace (all)"=w674, "time interval"=w683, "trace name"=w681, "database URL"=w684) -> ("error out"=w678:errorcluster, "quality"=w679:i32[], "historical trace"=w680:cluster{"timestamps":timestamp[], "data":dbl[]})  [unwired: 2 in, 1 out]
                }
                "Array 2" <- w663
                "Array" <- w662
              }
              frame Enabled {
                n294 = disable-structure shown="Disabled" {
                  disable-tunnel: w698 -> [w707 _]
                  disable-tunnel: w697 -> [w706 _]
                  disable-tunnel: [w705 _] -> w696
                  frame Disabled {
                    n295 = for {
                      tunnel: w707 -> [w712]
                      tunnel: w706 -> [w710] mode=indexing
                      tunnel: [w709] -> w705
                      n296 = call <vilib>:"Get Trace Info.vi"("timeout (30 s)"=1, "trace name"=w710, "database URL"=w712) -> ("error out"=w709:errorcluster, "first timestamp"=w708:timestamp)  [unwired: 4 in, 3 out]
                      n297 = To Double Precision Float(number=w708) -> ()  [unwired: 1 out]
                    }
                  }
                  frame Enabled {
                  }
                }
                n298 = call-poly <vilib>:"Read Traces.vi"("options"=w702, "timeout (30 s)"=w700, "max points per trace (all)"=w701, "error in (no error)"=w696, "time interval"=w704, "trace names"=w697, "database URL"=w698) -> ("error out"=w703:errorcluster, "quality"=w695:i32[][], "historical traces"=w699:T5)  [unwired: 1 in, 1 out]
                n299 = Empty Array?(array=w695) -> (empty?=w694:bool)
              }
            }
            "quality" <- w638
            "error out" <- w637
            "empty?" <- w630
            n300 = Bundle By Name(cluster=w643, "historical traces"=w634) -> (w642:T9)
            n301 = Format Into String(format string="Plot: Display Data>>%s", w626) -> (resulting string=w625:string)  [unwired: 2 in, 1 out]
            n302 = for {
              tunnel: w637 -> [w721]
              tunnel: w634 -> [_] mode=indexing
              n303 = call <vilib>:"Clear Errors.vi"("error in (no error)"=w721) -> ()  [unwired: 5 in, 2 out]
            }
            n304 = call <vilib>:"Clear Errors.vi"("error in (no error)"=w644) -> ("error out"=w641:errorcluster)  [unwired: 5 in, 1 out]
            "busy" <- TRUE ("Boolean")
          }
          frame True {
          }
        }
        n305 = call <userlib>:"Tick Count (ms)__ogtk.vi"("error in (no error)"=w611) -> ("error out"=w609:errorcluster, "millisecond timer value"=w610:u32)  [unwired: 9 in]
        n306 = Subtract(x=w610, y=w608) -> (x-y=w607:u32)
        n307 = Divide(x=w607, y=u32 1000 ("x")) -> (x/y=→"time (s)":dbl)
        n308 = call <vilib>:"Add State(s) to Queue__jki_lib_state_machine.vi"("State(s) in Front (\"\")"=w616, "State(s) in (\"\")"=w623) -> ("States Out"=w622:string)  [unwired: 13 in]
      }
      frame "Plot: Display Data" {
        n309 = Unbundle By Name(w730) -> ("historical traces"=→"XY Graph":T5, "Traces"=w725:T2)
        n310 = local write "busy"(FALSE ("Boolean")) -> ()
        n311 = case shown="\"preset\"" w726 {
          tunnel: w725 -> [_ w734]
          tunnel: ["Traces: update cluster" ("State(s) in Front (\"\")") "" ("State(s) in Front (\"\")")] -> w724
          frame "False", Default {
          }
          frame "preset" {
            n312 = for {
              tunnel: w734 -> [w739] mode=indexing
              i -> [w740]
              (unwired) u8 2 ("Y Scale.Scale Fit")
              n313 = control-ref of="XY Graph"() -> (w741:refnum<vi>)
              n314 = Unbundle By Name(w739) -> ("L/R scale"=w745:bool, "Color Box"=w738:u32)
              n315 = To Unsigned Long Integer(number=w740) -> (unsigned 32bit integer=w742:u32)
              n316 = Select(t=u32 1 ("f"), s=w745, f=u32 0) -> (s? t:f=w737:u32)
              n317 = property class="XYGraph (strict)"(reference=w741, "Active Plot"=w742, "Plot.YScaleIdx"=w737, "Plot.Plot Color"=w738, "ActYScl"=w737, "YScale.ScaleFit"=u8 2 ("Y Scale.Scale Fit")) -> ()  [unwired: 1 in, 2 out]
            }
          }
        }
        n318 = call <vilib>:"Add State(s) to Queue__jki_lib_state_machine.vi"("State(s) in Front (\"\")"=w724, "State(s) in (\"\")"=w732) -> ("States Out"=w731:string)  [unwired: 13 in]
      }
      frame "csv export" {
        n319 = Unbundle By Name(w747) -> ()  [unwired: 1 out]
        n320 = call <vilib>:"Add State(s) to Queue__jki_lib_state_machine.vi"("State(s) in (\"\")"=w749) -> ("States Out"=w748:string)  [unwired: 14 in]
      }
      frame "Plot: Display Current" {
        n321 = Get Date/Time In Seconds() -> (seconds since 1Jan1904=w756:timestamp)
        n322 = property on="Time slots" class="Enum (strict)"(error in=w753) -> (error out=w754:errorcluster, "Value"=w755:T3)  [unwired: 1 in, 1 out]
        n323 = property on="Time slots" class="Enum (strict)"(error in=w754, "Val(Sgnl)"=w755) -> (error out=w752:errorcluster)  [unwired: 1 in, 1 out]
        n324 = Bundle By Name(cluster=w758, "time interval.stop timestamp (now)"=w756, "Display Current Enable"=TRUE) -> (w757:T9)
        n325 = call <vilib>:"Add State(s) to Queue__jki_lib_state_machine.vi"("State(s) in Front (\"\")"="Plot: Calculate interpolation interval" ("State(s) in Front (\"\")"), "State(s) in (\"\")"=w760) -> ("States Out"=w759:string)  [unwired: 13 in]
      }
      frame "Plot: clear" {
        n326 = invoke on="Tree" class="Tree (strict)" method="Reinit To Default"(error in=w762) -> (error out=w761:errorcluster)  [unwired: 2 in, 2 out]
        n327 = property on="Time slots" class="Enum (strict)"(error in=w761) -> (error out=w767:errorcluster, "Value"=w768:T3)  [unwired: 1 in, 1 out]
        n328 = property on="Time slots" class="Enum (strict)"(error in=w767, "Val(Sgnl)"=w768) -> (error out=w766:errorcluster)  [unwired: 1 in, 1 out]
        n329 = Bundle By Name(cluster=w765, "Trace Names"=string[] []) -> (w764:T9)
        n330 = call <vilib>:"Add State(s) to Queue__jki_lib_state_machine.vi"("State(s) in (\"\")"=w770) -> ("States Out"=w769:string)  [unwired: 14 in]
      }
    }
  }
